vi "_FPGA_Aux_Reg_Scale&Amp.vi"(0 "Data in":u64) -> ()   [LabVIEW 2018]
uses:
  <vilib>/rvi/Emulation/niFpgaEmulationIsFPGAContextNoSignature.vi
  <vilib>/rvi/DataTransferAndStorage/Container/Common/niFpgaContainerGetUniqueNameForEmu.vi
  <vilib>/rvi/Memory/Memory_Emulation/niFpgaMemoryEmulationCacheClearOnFirstRun.vi
  <vilib>/rvi/Memory/Memory_Emulation/nirvimemoryEmulationManagerCache_MakeExclusive.vi
  <vilib>/rvi/Memory/Memory_Emulation/niFpgaMemoryEmulationValidateCache.vi
  <vilib>/rvi/Memory/Memory_Emulation/nirvimemoryEmulationManagerCache_InsertValue.vi
  <vilib>/Utility/error.llb/Clear Errors.vi
  <vilib>/rvi/Memory/Memory_Emulation/nirvimemoryEmulationManagerCache_ReleaseExclusive.vi
  <vilib>/rvi/Memory/Memory_Emulation/nirvimemoryEmulationManagerCache_GetValue.vi
  <vilib>/rvi/Memory/Memory_Emulation/nirvimemoryEmulationManagerCache_SetValue.vi
  <vilib>/rvi/Emulation/niFpgaProcessEmulError.vi
  <vilib>/rvi/Emulation/niFpgaSctlEmulationGetInTimedLoop.vi
  <vilib>/rvi/DataTransferAndStorage/Container/XNode/niFpgaContainer.xnode
  <vilib>/rvi/DataTransferAndStorage/Register/Emulation/niFpgaRegisterEmulation.vi
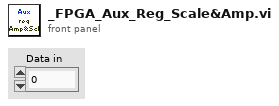
[diagram p1: front panel]
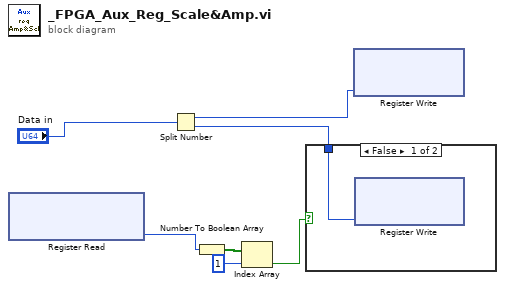
[diagram p0: block diagram]
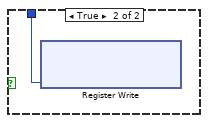
[diagram p2: hidden frame]
diagram:
  n1 = xnode "Register Read"() -> ("Data"=w5:u8)  [unwired: 1 in, 1 out]
  n2 = Split Number(x="Data in") -> (hi(x)=w7:u32, lo(x)=w2:u32)
  n3 = Number To Boolean Array(number=w5) -> (Boolean array=w3:bool[])
  n4 = Index Array(array=w3, index=1) -> (element=w6:bool)
  n5 = case shown="False" w6 {
    tunnel: w2 -> [w8 w9]
    frame False {
      n6 = xnode "Register Write"("Data"=w8) -> ()  [unwired: 1 in, 1 out]
    }
    frame True {
      n7 = xnode "Register Write"("Data"=w9) -> ()  [unwired: 1 in, 1 out]
    }
  }
  n8 = xnode "Register Write"("Data"=w7) -> ()  [unwired: 1 in, 1 out]
